vi "Append Digital Data By Signal.vi"() -> ()   [LabVIEW 2023]
doc: "This example illustrates how to append separate digital signals into one Digital Waveform.\n\nThe front panel has three digital controls that can be interactively edited by the user. The combined signals are displayed both numerically and graphically."
uses:
  <vilib>/Waveform/DTblOps.llb/DTbl Append Digital Signals.vi
panel:
  out "Digital Waveform Graph":digitaldata(graph)
  out "Digital Data Output":digitaldata
  in  "Digital Data 3":digitaldata={"transitions"=[], "data"=[[0, 0, 0, 0, 1, 1], [0, 0, 1, 0, 0, 1], [1, 0, 1, 0, 1, 0]]}
  in  "Digital Data 2":digitaldata={"transitions"=[], "data"=[[0, 0, 0, 0, 1, 0], [0, 0, 0, 1, 0, 1], [1, 0, 1, 0, 1, 0]]}
  in  "Digital Data 1":digitaldata={"transitions"=[], "data"=[[0, 0, 0, 0, 1], [0, 0, 1, 0, 0], [1, 0, 1, 0, 1]]}
  # "Overview: Illustrates how to append separate digital signals into a single value.\nInstructions:\nRun the VI."
  # "The values of Digital Data 1, Digital Data 2, and Digital Data 3 are appended by signal, then displayed in the Digital Data Output and Digital Waveform Graph indicators."
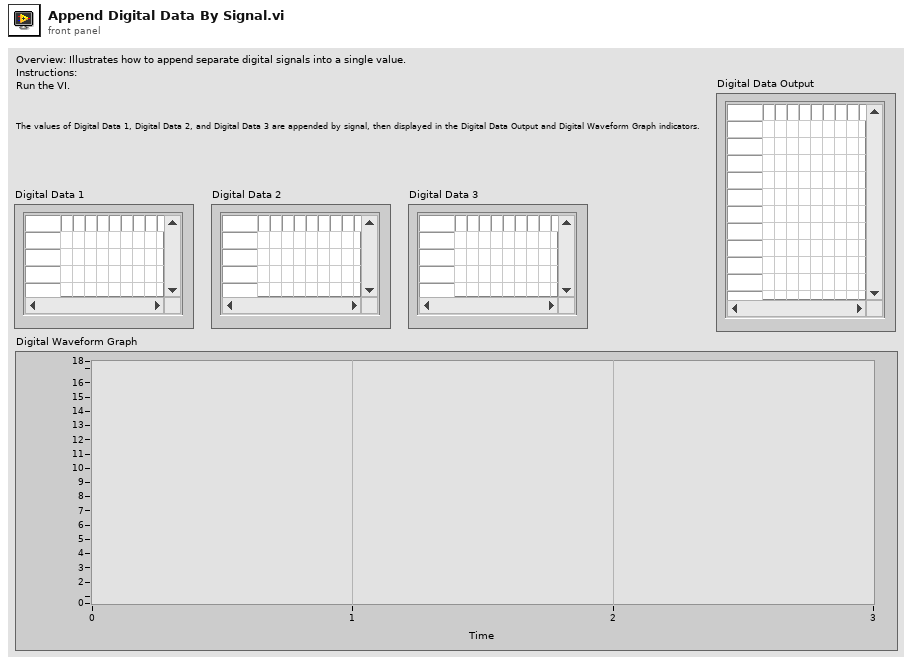
[diagram p1: front panel]
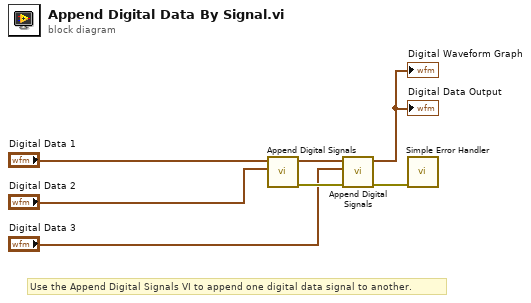
[diagram p0: block diagram]
diagram:
  # "Use the Append Digital Signals VI to append one digital data signal to another."
  n1 = call-poly <vilib>:"Append Digital Signals.vi"("digital data (low bits)"="Digital Data 2", "digital data (high bits)"="Digital Data 1") -> ("error out"=w7:errorcluster, "digital data out"=w4:digitaldata)  [unwired: 8 in]
  n2 = call-poly <vilib>:"Append Digital Signals.vi"("error in (no error)"=w7, "digital data (low bits)"="Digital Data 3", "digital data (high bits)"=w4) -> ("error out"=w6:errorcluster, "digital data out"=→"Digital Data Output" →"Digital Waveform Graph":digitaldata)  [unwired: 7 in]
  n3 = call <vilib>:"Simple Error Handler.vi"("error in (no error)"=w6) -> ()  [unwired: 4 in, 5 out]
